vi "ZCAN_ReadChannelErrInfo.vi"(1 "can_index_handle":u64, 3 "error in (no error)":errorcluster caption="错误输入（无错误）") -> (6 "ChannelErrInfo(string out)":string, 8 "error out":errorcluster caption="错误输出")   [LabVIEW 2018, in "zlgcan.lvlib"]
doc: "该函数用于读取通道的错误信息。"
uses:
  zlgcan.lvlib
  data_type/ZCAN_CHANNEL_ERROR_INFO.ctl
  bin/ControlCANFD.dll
panel:
  out "pErrInfo":T1
  in  "ZCAN_CHANNEL_ERROR_INFO(in)":T1
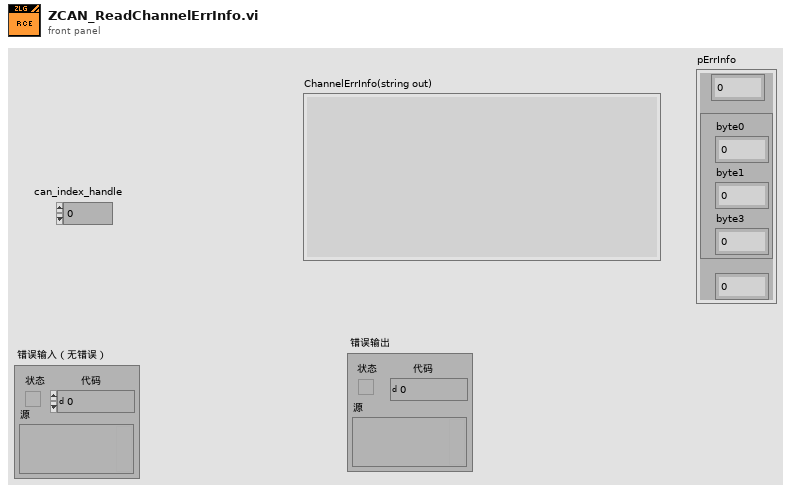
[diagram p1: front panel]
types:
  T1 = typedef "ZCAN_CHANNEL_ERROR_INFO.ctl" = cluster{"error_code":u32, "passive_ErrData":cluster{"byte0":u8, "byte1":u8, "byte3":u8}, "arLost_ErrData":u8}
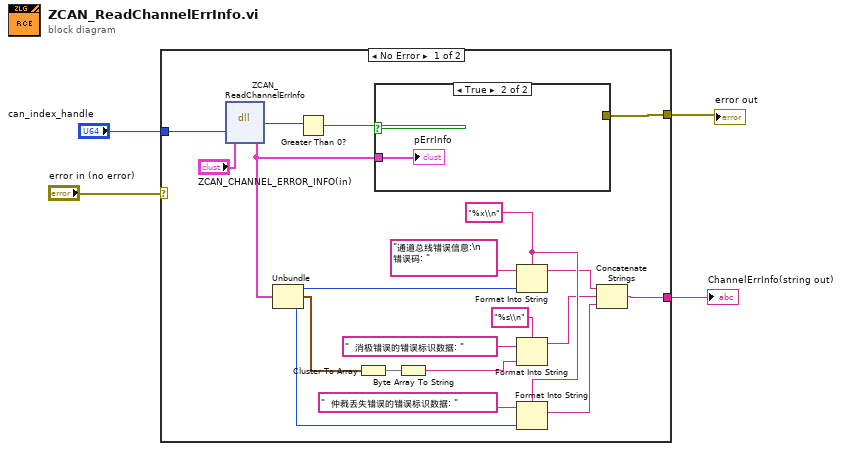
[diagram p0: block diagram]
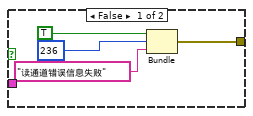
[diagram p2: hidden frame]
diagram:
  n1 = case shown="No Error" "error in (no error)" {
    selector: "error in (no error)" -> [_ w30]
    tunnel: [w21 w30] -> w2
    tunnel: "can_index_handle" -> [w24 _]
    tunnel: [w11 _] -> w1
    frame No Error {
      w12 = "%x\\n" ("format string")
      n2 = dll-call lib="C:/Users/ttc52/Desktop/DHC FD LV2018/LABIVIEW CANFD Tool_V1.2.4_20220724/bin/ControlCANFD.dll" fn="ZCAN_ReadChannelErrInfo"("channel_handle"=w24, "pErrInfo"="ZCAN_CHANNEL_ERROR_INFO(in)") -> ("return"=w23:u32, "pErrInfo"=w5:T1)  [unwired: 4 in, 2 out]
      n3 = Unbundle(w5) -> ("error_code"=w13:u32, "passive_ErrData"=w16:cluster{"byte0":u8, "byte1":u8, "byte3":u8}, "arLost_ErrData"=w8:u8)
      n4 = Greater Than 0?(x=w23) -> (x > 0?=w22:bool)
      n5 = Cluster To Array(cluster=w16) -> (array=w15:u8[])
      n6 = case shown="True" w22 {
        tunnel: [w25 _] -> w21
        tunnel: w5 -> [_ w29]
        frame False {
          n7 = Bundle("status"=TRUE, "code"=236, "消息"="读通道错误信息失败") -> (w25:cluster{"status":bool, "code":i32, "消息":string})  [unwired: 1 in]
        }
        frame True {
          "pErrInfo" <- w29
        }
      }
      n8 = Byte Array To String(unsigned byte array=w15) -> (string=w14:string)
      n9 = Format Into String(format string=w12, initial string="通道总线错误信息:\n  错误码: ", w13) -> (resulting string=w10:string)  [unwired: 1 in, 1 out]
      n10 = Format Into String(format string="%s\\n", initial string="  消极错误的错误标识数据: ", w14) -> (resulting string=w9:string)  [unwired: 1 in, 1 out]
      n11 = Format Into String(format string=w12, initial string="  仲裁丢失错误的错误标识数据: ", w8) -> (resulting string=w7:string)  [unwired: 1 in, 1 out]
      n12 = Concatenate Strings(w10, w9, w7) -> (w11:string)
    }
    frame Error {
    }
  }
  "error out" <- w2
  "ChannelErrInfo(string out)" <- w1
